vi "PAN_MacroCheckPath.vi"(10 "CommandStr":string, 11 "macrodir":path) -> (0 "error out":errorcluster, 2 "dir?":bool, 3 "output path":path)   [LabVIEW 2016]
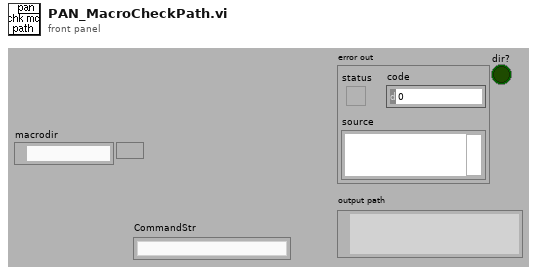
[diagram p1: front panel]
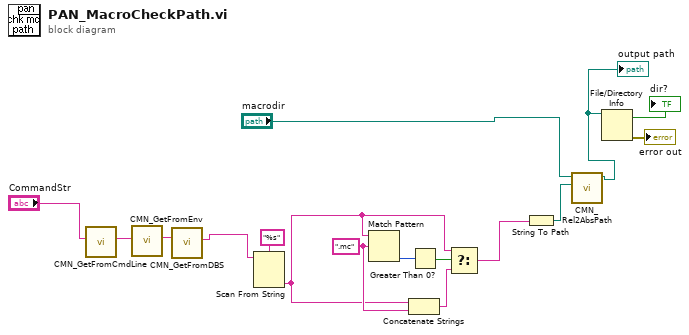
[diagram p0: block diagram]
diagram:
  w10 = ".mc" ("regular expression")
  n1 = call "CMN_GetFromCmdLine.vi"("str in"="CommandStr") -> ("str out"=w3:string)  [unwired: 10 out]
  n2 = call "CMN_GetFromEnv.vi"("str in"=w3) -> ("str out"=w4:string)  [unwired: 10 out]
  n3 = call "CMN_GetFromDBS.vi"("str in"=w4) -> ("str out"=w1:string)  [unwired: 10 out]
  n4 = Scan From String(format string="%s", input string=w1) -> (output 1=w5:string)  [unwired: 2 in, 4 out]
  n5 = Match Pattern(string=w5, regular expression=w10) -> (offset past match=w14:i32)  [unwired: 4 out]
  n6 = Concatenate Strings(w5, w10) -> (w11:string)
  n7 = Greater Than 0?(x=w14) -> (x > 0?=w13:bool)
  n8 = Select(t=w5, s=w13, f=w11) -> (s? t:f=w12:string)
  n9 = String To Path(string=w12) -> (path=w16:path)
  n10 = call "CMN_Rel2AbsPath.vi"("test path"=w16, "absolute path"="macrodir") -> ("output path"=w15:path)  [unwired: 1 in, 8 out]
  "output path" <- w15
  n11 = File/Directory Info(path=w15) -> (directory=→"dir?":bool, error out=→"error out":errorcluster)  [unwired: 1 in, 5 out]
